vi "Configure Power on Setup.vi"(8 "error in (no error)":errorcluster, 11 "VISA resource name":refnum<visa-resource-name>) -> (0 "error out":errorcluster, 3 "VISA resource name out":refnum<visa-resource-name>)   [LabVIEW 2016, in "Keithley DMM7510.lvlib"]
doc: "This VI selects the defaults that are used when you power on the instrument."
uses:
  Keithley DMM7510.lvlib
panel:
  in  "Setup":u16(ring) items=["Default", "Setup 0", "Setup 1", "Setup 2", "Setup 3", "Setup 4"]
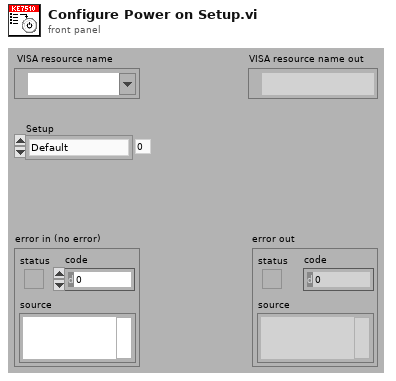
[diagram p1: front panel]
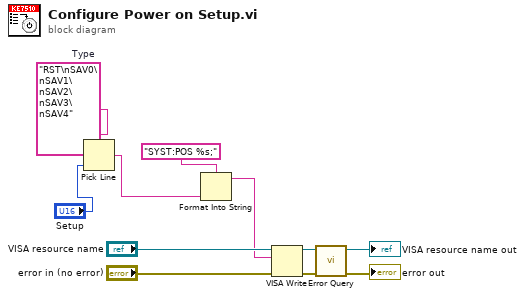
[diagram p0: block diagram]
diagram:
  w3 = "RST\nSAV0\nSAV1\nSAV2\nSAV3\nSAV4"  # Type
  n1 = Pick Line(multi-line string=w3, line index="Setup") -> (output string=w1:string)  [unwired: 1 in]
  n2 = Format Into String(format string="SYST:POS %s;", w1) -> (resulting string=w5:string)  [unwired: 2 in, 1 out]
  n3 = VISA Write(VISA resource name="VISA resource name", write buffer=w5, error in (no error)="error in (no error)") -> (VISA resource name out=w7:refnum<visa-resource-name>, error out=w6:errorcluster)  [unwired: 1 out]
  n4 = call "Error Query.vi"("error in (no error)"=w6, "VISA resource name"=w7) -> ("error out"=→"error out":errorcluster, "VISA resource name out"=→"VISA resource name out":refnum<visa-resource-name>)  [unwired: 8 out]
